vi "Draw Textured Triangle v3.vi"(0 "Texture 3":T2={"x"=1.0, "y"=0.0} {"y" min=0 max=1 step=0.1; "x" min=0 max=1 step=0.1}, 4 "Texture 2":T2={"x"=0.0, "y"=1.0} {"y" min=0 max=1 step=0.1; "x" min=0 max=1 step=0.1}, 8 "Point 3":T3={"x"=256, "y"=512}, 9 "Point 2":T3={"x"=512, "y"=256}, 10 "Point 1":T3) -> ()   [LabVIEW 2022 SP3, in "Raster.lvlib"]
uses:
  Raster.lvlib
  Point 2D.ctl
  Point 2D (SGL).ctl
  <vilib>/Utility/miscctls.llb/LVPointTypeDef.ctl
  Screen Dimensions.ctl
  Utility/Convert Pixels To Picture.vi/d601d993-a776-4dc8-89c7-357d8398c88c.vi
  Utility/Convert Pixels To Picture.vi/7816d0d6-8e4d-41a2-85ac-ed82f1435763.vi
  <vilib>/Utility/High Resolution Relative Seconds.vi
  <vilib>/picture/picture.llb/Draw Unflattened Pixmap.vi
  <vilib>/picture/picture.llb/Draw True-Color Pixmap.vi
  Utility/Utility.lvlib
panel:
  in  "Origin":T1={"Horizontal"=0, "Vertical"=486}
  in  "24-bit pixmap":u32[][](array[numeric]) format="%x"
  in  "Texture 1":T2={"x"=1.0, "y"=1.0} {"y" min=0 max=1 step=0.1; "x" min=0 max=1 step=0.1}
  in  "Path":path=path "C:/dev/3DEngine/Resource/Models/Textured Plane Base Colour.png"
  out "2D Picture 2":picture
  # "Not working"
  # "Not working"
  # "(0,1)"
  # "(1,1)"
  # "(0,0)"
  # "(1,0)"
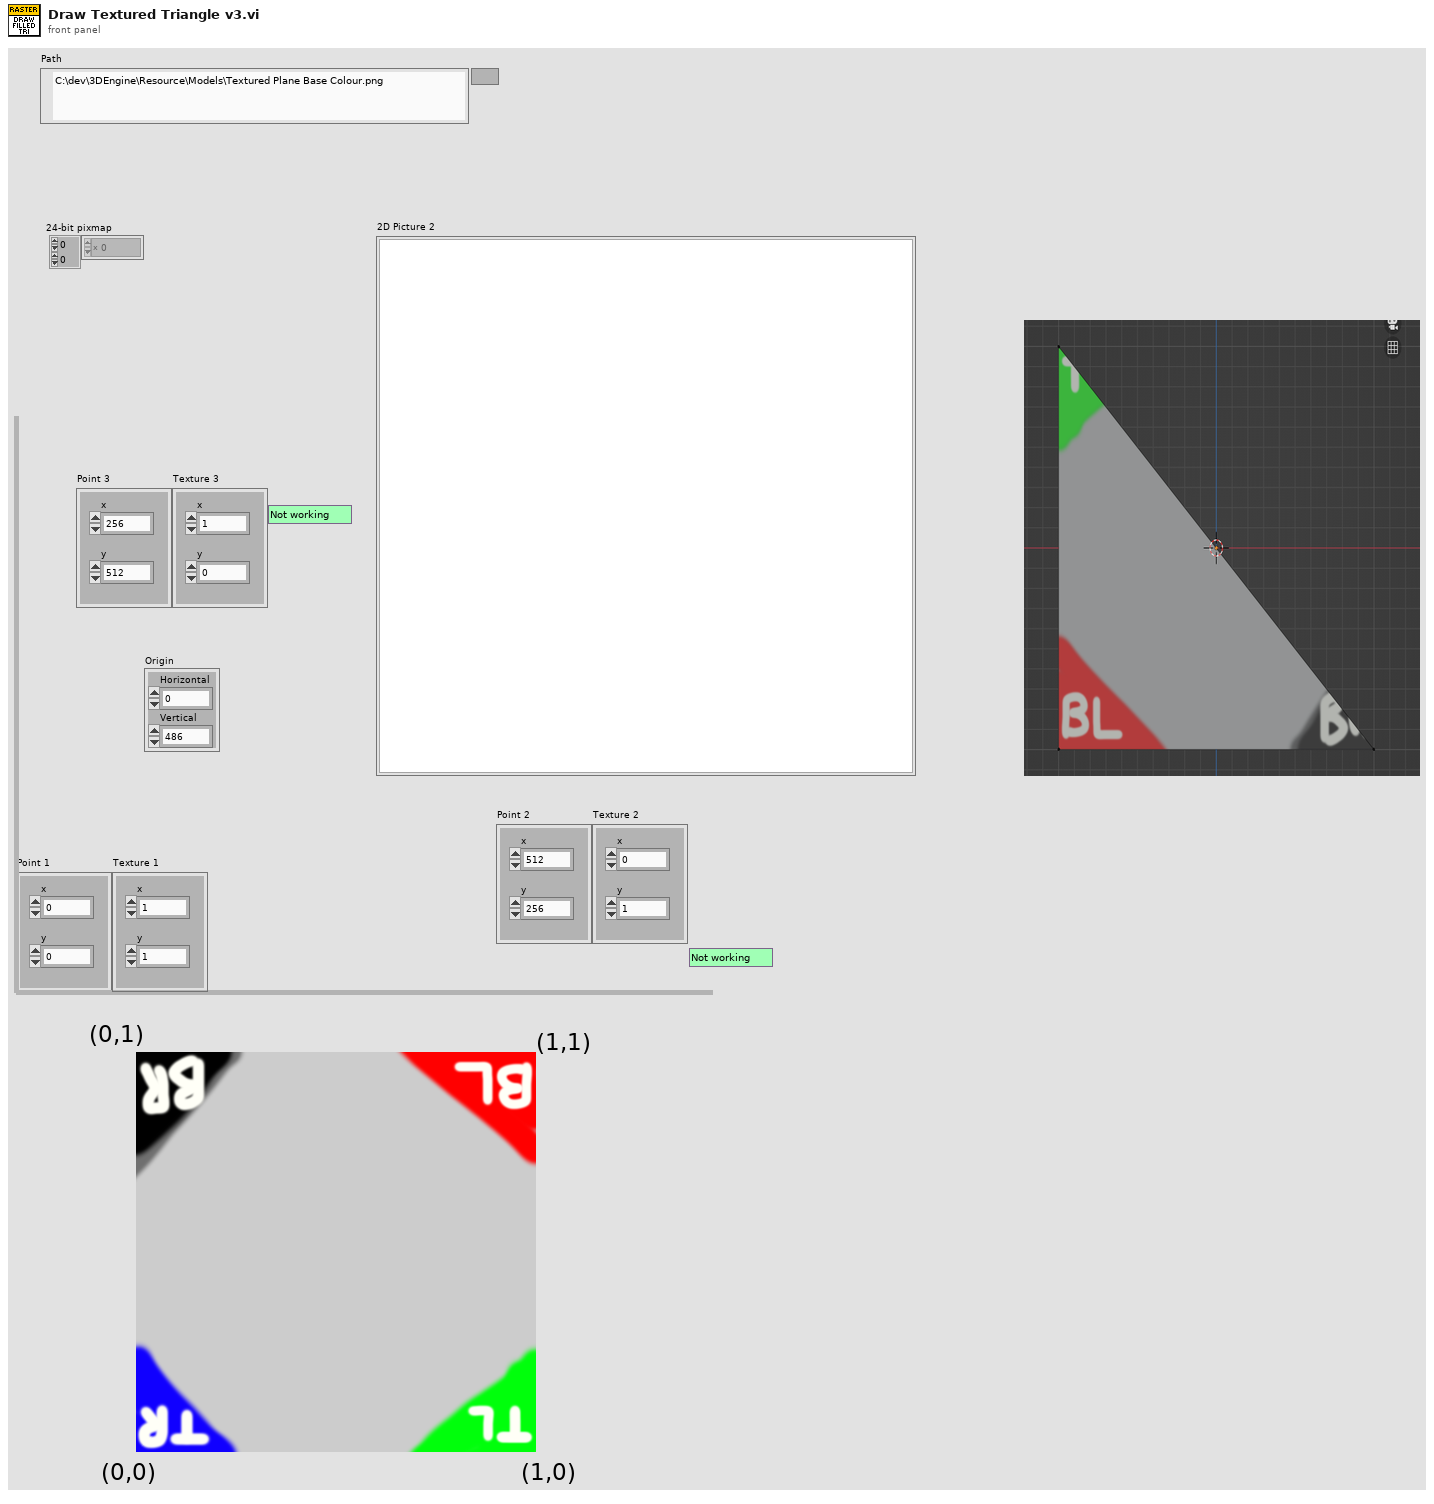
[diagram p1: front panel]
types:
  T1 = typedef "LVPointTypeDef.ctl" = cluster{"Horizontal":i16, "Vertical":i16}
  T2 = typedef "Raster.lvlib/Point 2D (SGL).ctl" = cluster{"x":sgl, "y":sgl}
  T3 = typedef "Raster.lvlib/Point 2D.ctl" = cluster{"x":i32, "y":i32}
  T4 = typedef "Raster.lvlib/Screen Dimensions.ctl" = cluster{"Width":u32, "Height":u32}
  T5 = typedef "imagedata.ctl" = cluster{"image type":i32, "image depth":i32, "image":u8[], "mask":u8[], "colors":u32[], "Rectangle":cluster{"left":i16, "top":i16, "right":i16, "bottom":i16}}
  T6 = cluster{"Texture 1":T2, "Texture 2":T2, "Texture 3":T2}
  T7 = cluster{"Texture 1":T3, "Texture 2":T3, "Texture 3":T3}
  T8 = typedef "Raster.lvlib/Line Parameters.ctl" = cluster{"1/m":sgl, "c":sgl}
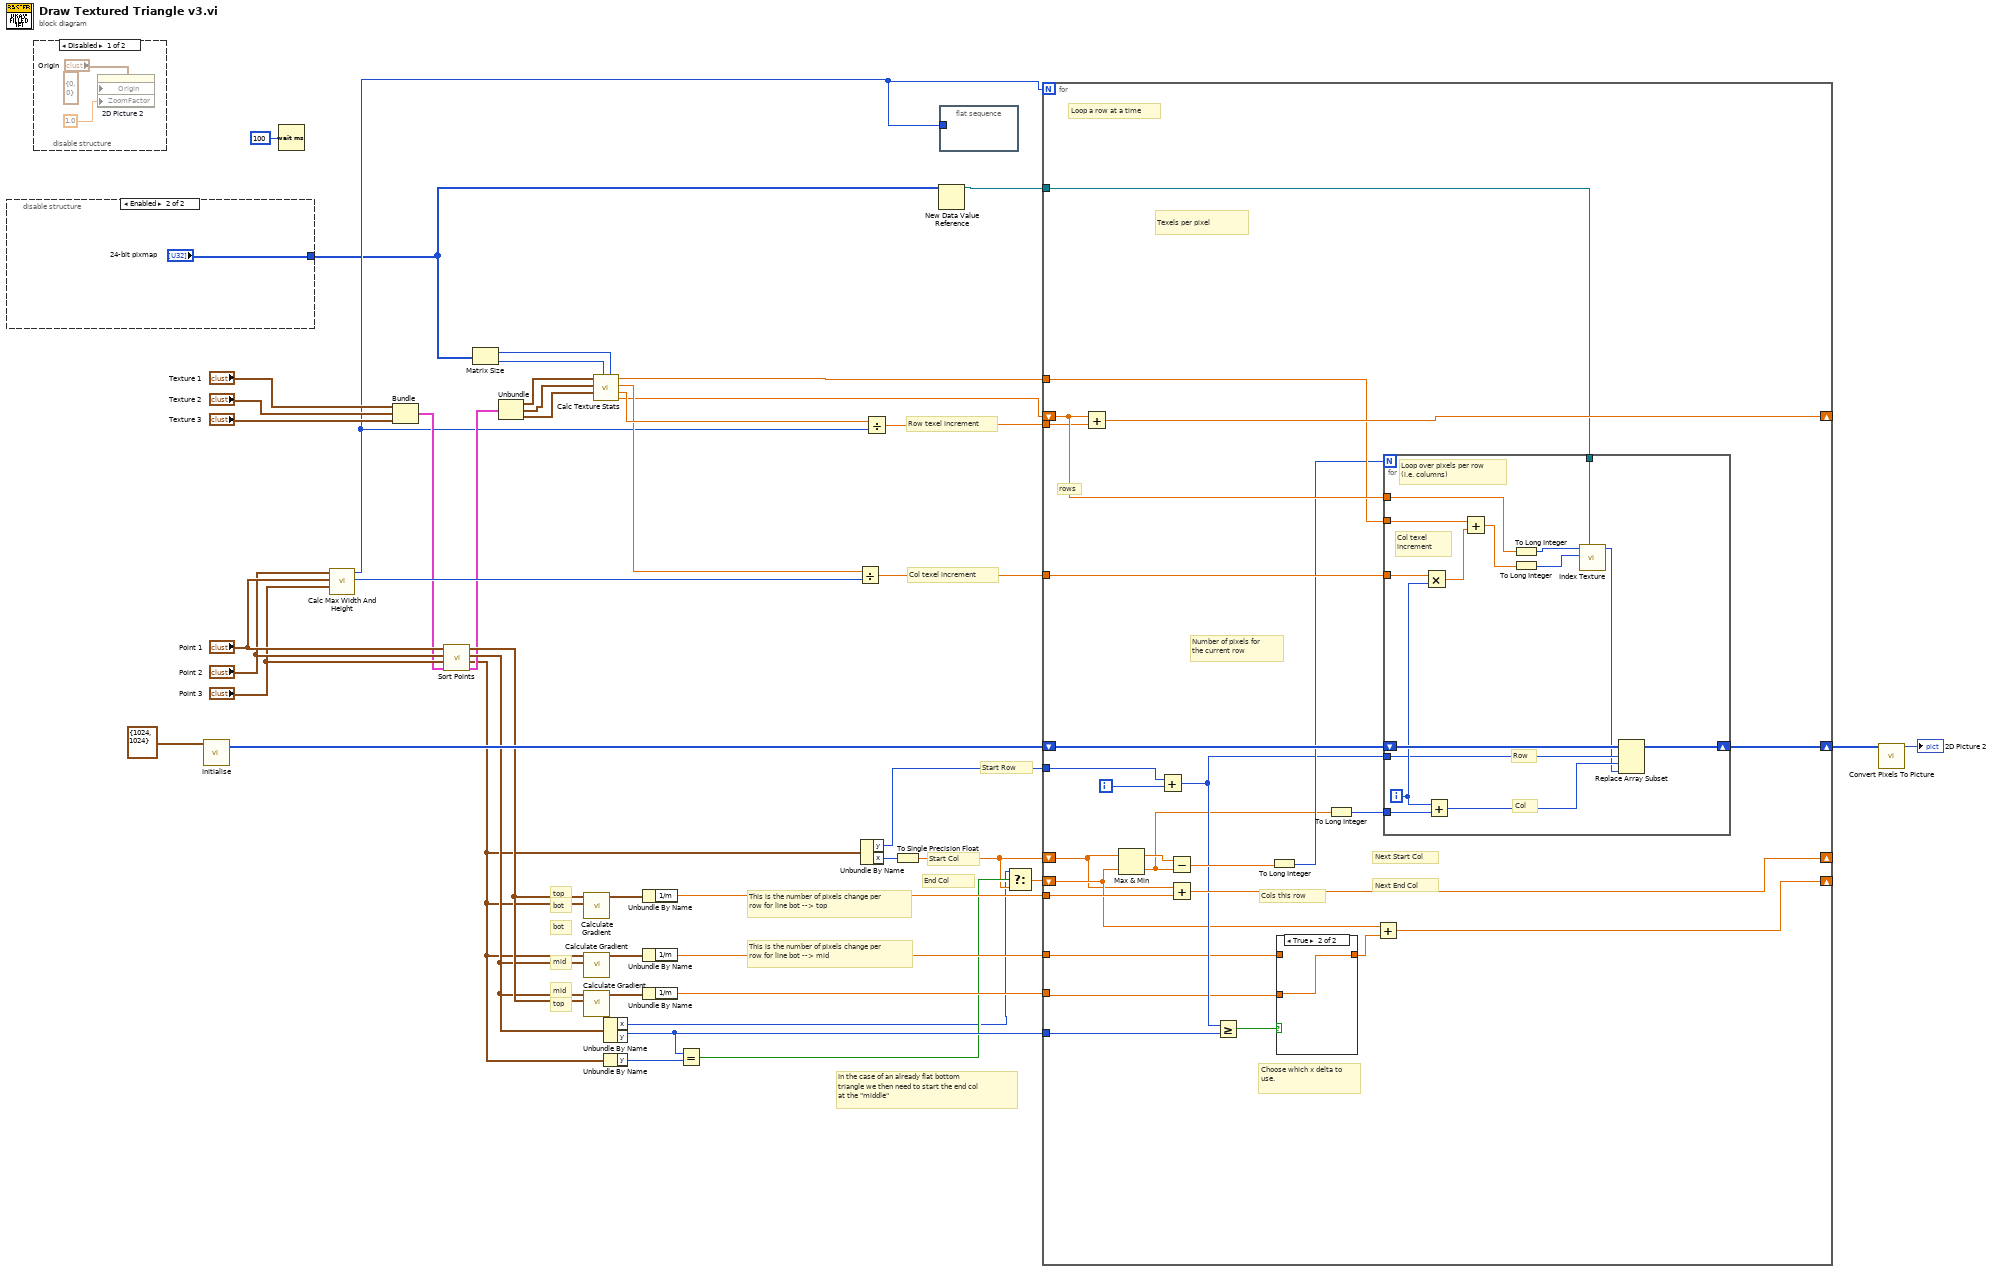
[diagram p0: block diagram]
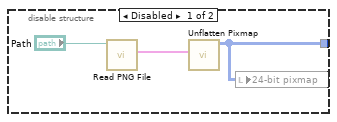
[diagram p3: hidden frame]
diagram:
  # "In the case of an already flat bottom triangle we then need to start the end col at the \"middle\""
  # "top"
  # "mid"
  # "mid"
  # "bot"
  # "bot"
  # "top"
  # "Row texel increment"
  # "Col texel increment"
  # "End Col"
  # "This is the number of pixels change per row for line bot --> top"
  # "This is the number of pixels change per row for line bot --> mid"
  # "Start Col"
  # "Start Row"
  n1 = disable-structure shown="Enabled" {
    disable-tunnel: [w46 "24-bit pixmap"] -> w11
    frame Disabled {
      n2 = call <vilib>:"Read PNG File.vi"("path to PNG file"="Path") -> ("image data"=w47:T5)  [unwired: 8 in, 2 out]
      n3 = call <vilib>:"Unflatten Pixmap.vi"("image data"=w47) -> ("24-bit pixmap"=w46:u32[][])  [unwired: 4 in, 6 out]
      n4 = local write "24-bit pixmap"(w46) -> ()
    }
    frame Enabled {
    }
  }
  n5 = disable-structure shown="Disabled" {
    frame Disabled {
      (unwired) T1 {"Horizontal"=0, "Vertical"=0} ("Origin")
      n6 = property on="2D Picture 2" class="Pict"("Origin"="Origin", "ZoomFactor"=sgl 1.0 ("Zoom Factor")) -> ()  [unwired: 2 in, 2 out]
    }
    frame Enabled {
    }
  }
  n7 = call "Initialise.vi"("Screen Dimensions"=T4 {"Width"=1024, "Height"=1024}) -> ("Pixel Data out"=w44:u32[][])  [unwired: 10 in]
  n8 = Wait (ms)(milliseconds to wait=u32 100) -> ()  [unwired: 1 out]
  n9 = call "Calc Max Width And Height.vi"("Point 3"="Point 3", "Point 2"="Point 1", "Point 1"="Point 2") -> ("Max Width"=w39:i32, "Max Height"=w12:i32)  [unwired: 7 in]
  n10 = Bundle("Texture 1"="Texture 1", "Texture 2"="Texture 2", "Texture 3"="Texture 3") -> (w21:T6)  [unwired: 1 in]
  n11 = call "Sort Points.vi"("Texture Vertices"=w21, "Point 3"="Point 3", "Point 2"="Point 2", "Point 1"="Point 1") -> ("Texture Vertices 2"=w16:T7, "Bottom"=w7:T3, "Middle"=w17:T3, "Top"=w20:T3)  [unwired: 4 in]
  n12 = Matrix Size(0:w11) -> (1:w29:i32, 2:w28:i32)
  n13 = Unbundle(w16) -> ("Texture 1"=w15:T3, "Texture 2"=w14:T3, "Texture 3"=w13:T3)
  n14 = call "Calculate Gradient.vi"("P2"=w7, "P1"=w20) -> ("Line Parameters"=w33:T8)  [unwired: 9 in]
  n15 = call "Calculate Gradient.vi"("P2"=w17, "P1"=w7) -> ("Line Parameters"=w37:T8)  [unwired: 9 in]
  n16 = call "Calculate Gradient.vi"("P2"=w20, "P1"=w17) -> ("Line Parameters"=w19:T8)  [unwired: 9 in]
  n17 = call "Calc Texture Stats.vi"("Texture Number Of Rows"=w29, "Texture Number Of Cols"=w28, "Bottom"=w13, "Middle"=w14, "Top"=w15) -> ("Texel Start Row (v)"=w30:sgl, "Texels In Highest Col (v)"=w42:sgl, "Texels In Widest Row (u)"=w41:sgl, "Texel Start Col (u)"=w38:sgl)  [unwired: 3 in]
  n18 = Unbundle By Name(w17) -> ("x"=w2:i32, "y"=w6:i32)
  n19 = Unbundle By Name(w7) -> ("y"=w5:i32)
  n20 = Unbundle By Name(w33) -> ("1/m"=w32:sgl)
  n21 = Unbundle By Name(w37) -> ("1/m"=w36:sgl)
  n22 = Unbundle By Name(w19) -> ("1/m"=w18:sgl)
  n23 = Equal?(x=w6, y=w5) -> (x = y?=w4:bool)
  n24 = Divide(x=w41, y=w39) -> (x/y=w40:sgl)
  n25 = Unbundle By Name(w7) -> ("y"=w35:i32, "x"=w34:i32)
  n26 = Divide(x=w42, y=w12) -> (x/y=w43:sgl)
  n27 = To Single Precision Float(number=w34) -> (single precision float=w3:sgl)
  n28 = New Data Value Reference(data value=w11) -> (data value reference=w10:refnum<data-value>)  [unwired: 1 in, 1 out]
  n29 = flat-sequence {
    tunnel: w12 -> [_]
    frame #0 {
    }
  }
  n30 = Select(t=w2, s=w4, f=w3) -> (s? t:f=w1:sgl)
  n31 = for {
    N: w12 -> [_]
    shift-right: [w76] -> w8
    shift-left: w44 -> [w77]
    tunnel: w10 -> [w70]
    shift-right: [w74] -> _
    shift-left: w30 -> [w75]
    tunnel: w43 -> [w73]
    tunnel: w38 -> [w72]
    tunnel: w40 -> [w71]
    tunnel: w36 -> [w59]
    tunnel: w35 -> [w63]
    shift-right: [w68] -> _
    shift-left: w3 -> [w54]
    shift-right: [w67] -> _
    shift-left: w1 -> [w56]
    tunnel: w32 -> [w69]
    tunnel: w18 -> [w57]
    tunnel: w6 -> [w60]
    i -> [w62]
    # "Choose which x delta to use."
    # "Loop a row at a time"
    # "Cols this row"
    # "Next End Col"
    # "Next Start Col"
    # "Texels per pixel"
    # "Number of pixels for the current row"
    # "rows"
    n32 = Add(x=w75, y=w73) -> (x+y=w74:sgl)
    n33 = Max & Min(x=w54, y=w56) -> (max(x,y)=w55:sgl, min(x,y)=w53:sgl)
    n34 = Add(x=w63, y=w62) -> (x+y=w61:i32)
    n35 = Subtract(x=w55, y=w53) -> (x-y=w65:sgl)
    n36 = Add(x=w54, y=w69) -> (x+y=w68:sgl)
    n37 = Greater Or Equal?(x=w61, y=w60) -> (x >= y?=w52:bool)
    n38 = To Long Integer(number=w65) -> (32bit integer=w64:i32)
    n39 = case shown="True" w52 {
      tunnel: w59 -> [w78 _]
      tunnel: [w78 w79] -> w58
      tunnel: w57 -> [_ w79]
      frame False {
      }
      frame True {
      }
    }
    n40 = To Long Integer(number=w53) -> (32bit integer=w66:i32)
    n41 = Add(x=w56, y=w58) -> (x+y=w67:sgl)
    n42 = for {
      N: w64 -> [_]
      shift-right: [w80] -> w76
      shift-left: w77 -> [w94]
      tunnel: w75 -> [w92]
      tunnel: w72 -> [w91]
      tunnel: w71 -> [w90]
      tunnel: w70 -> [w84]
      tunnel: w66 -> [w88]
      tunnel: w61 -> [w85]
      i -> [w87]
      # "Loop over pixels per row (i.e. columns)"
      # "Col texel increment"
      # "Col"
      # "Row"
      # "cols"
      n43 = Multiply(x=w90, y=w87) -> (x*y=w89:sgl)
      n44 = Add(x=w87, y=w88) -> (x+y=w86:i32)
      n45 = Add(x=w91, y=w89) -> (x+y=w93:sgl)
      n46 = To Long Integer(number=w92) -> (32bit integer=w83:i32)
      n47 = To Long Integer(number=w93) -> (32bit integer=w82:i32)
      n48 = call "Index Texture.vi"("data value reference"=w84, "Col Index"=w82, "Row Index"=w83) -> ("Colour"=w81:u32)  [unwired: 8 in]
      n49 = Replace Array Subset(array=w94, new element=w81, index (row)=w85, index (col)=w86) -> (w80:u32[][])
    }
  }
  n50 = call "Convert Pixels To Picture.vi"("Pixel Data in"=w8) -> ("2D Picture"=→"2D Picture 2":picture)  [unwired: 9 in, 1 out]
